vi "cDAQ Voltage - Finite Output.vi"() -> ()   [LabVIEW 2019]
doc: "This example demonstrates how to generate a finite amount of data from a buffer in your computer's memory."
uses:
  <vilib>/Utility/error.llb/DialogType.ctl
  <vilib>/DAQmx/write.llb/DAQmx Write (Analog 1D Wfm NChan NSamp).vi
  <vilib>/DAQmx/read.llb/DAQmx Read (Analog 1D DBL 1Chan NSamp).vi
  <vilib>/DAQmx/create/channels.llb/DAQmx Create Channel (AO-Voltage-Basic).vi
  <vilib>/DAQmx/configure/timing.llb/DAQmx Timing (Sample Clock).vi
  <vilib>/DAQmx/configure/trigger.llb/DAQmx Start Trigger (Digital Edge).vi
  <vilib>/DAQmx/configure/trigger.llb/DAQmx Start Trigger (Time).vi
  <vilib>/DAQmx/configure/trigger.llb/DAQmx Start Trigger (Analog Edge).vi
  <vilib>/DAQmx/miscellaneous.llb/DAQmx Fill In Error Info.vi
  <vilib>/DAQmx/configure/events/hardwareSignals.llb/DAQmx Export Signal (Most Signals).vi
  <vilib>/DAQmx/create/channels.llb/DAQmx Create Channel (AI-Voltage-Basic).vi
  <resource>/objmgr/daqmx.rc
  <vilib>/measure/NI_MABase.lvlib
panel:
  out "Waveform Graph 2":dbl[](graph)
  in  "physical channels":tag="cDAQ1Mod1/ai0"
  in  "Trigger Type":T1(tab)
  in  "Digital Start Trigger Edge":i32(ring)=10280 caption="Edge" items=["Rising"=10280, "Falling"=10171]
  in  "Digital Start Trigger Source":tag="/Dev1/PFI0" caption="Source"
  in  "Digital Pause Trigger Pause When":i32(ring)=10192 caption="Pause When" items=["High"=10192, "Low"=10214]
  in  "Digital Pause Trigger Source":tag="/Dev1/PFI0" caption="Source"
  in  "Analog Start Trigger Level":dbl caption="Level" format="%0.2f"
  in  "Analog Start Trigger Hysteresis":dbl caption="Hysteresis" format="%.2f"
  in  "Analog Start Trigger Slope":i32(ring)=10280 caption="Slope" items=["Rising"=10280, "Falling"=10171]
  in  "Analog Start Trigger Source":string="APFI0" caption="Source"
  in  "Analog Pause Trigger Source":string="APFI0" caption="Source"
  in  "Analog Pause Trigger Pause When":i32(ring)=10093 caption="Pause When" items=["Above Level"=10093, "Below Level"=10107]
  in  "Analog Pause Trigger Level":dbl caption="Level" format="%.2f"
  in  "When":timestamp
  in  "Select Time\nManually":bool
  in  "Output Array":T2(array[cluster])=[{"Waveform Type"=0, "Amplitude"=1.0, "Frequency"=10.0}] {"Frequency" format="%0.2p"; "Amplitude" format="%0.2p"; "Waveform Type" items=["Sine Wave", "Triangle Wave", "Square Wave", "Sawtooth Wave"]}
  in  "Number of Samples":i32=1000
  out "Waveform Graph":waveform(dbl)[](graph)=[{"t0"=timestamp(0 s since 1904-01-01), "dt"=0.001, "Y"=array[1000 elements]}]
  in  "Sample Rate":dbl=1000.0
  in  "Sample Clock Source":tag="OnboardClock"
  in  "Max Voltage":dbl=5.0
  in  "Min Voltage":dbl=-5.0
  in  "Physical Channel(s)":tag="cDAQ1Mod2/ao0"
  out "Actual Sample Rate":dbl=1000.0 format="%0.2f"
  # "Channel Settings"
  # "Output"
  # "Timing and Buffer Settings"
  # "Waveform Settings"
  # "Trigger Settings"
  # "The number of elements in the waveform array\nmust equal the number of channels in the task."
  # "To enable triggers, select a tab above, and configure the settings.\n\nNot all hardware supports all trigger types. Refer to your device documentation for more information."
  # "This trigger type is not supported in output tasks. \n\nRefer to your device documentation for more information on which triggers are supported."
  # "This trigger type is not supported in output tasks. \n\nRefer to your device documentation for more information on which triggers are supported."
  # "If time is not manually set, task will begin after 10 seconds"
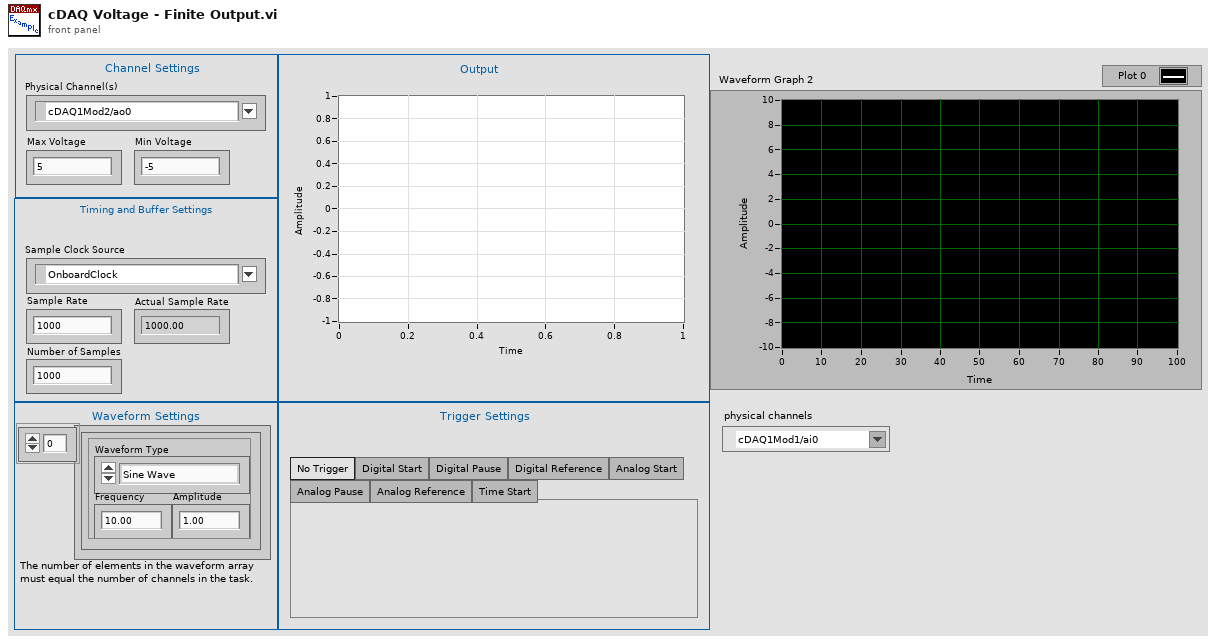
[diagram p1: front panel]
types:
  T1 = enum32{"No Trigger", "Digital Start", "Digital Pause", "Digital Reference", "Analog Start", "Analog Pause", "Analog Reference", "Time Start"}
  T2 = cluster{"Waveform Type":u16, "Amplitude":dbl, "Frequency":dbl}[]
  T3 = typedef "DialogType.ctl" = u16
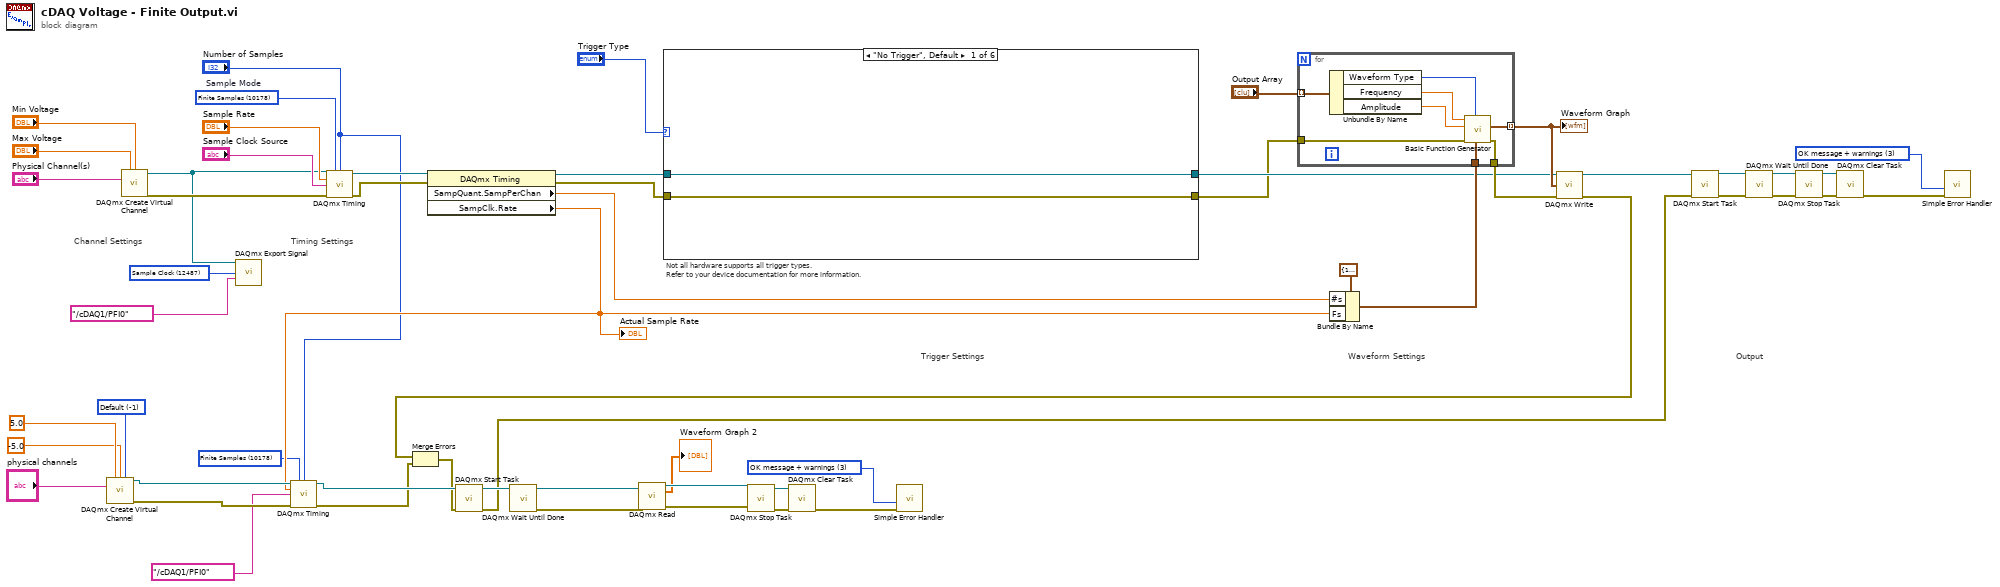
[diagram p0: block diagram]
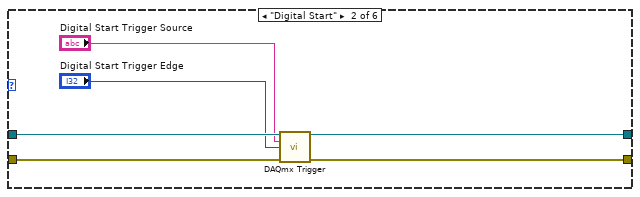
[diagram p2: hidden frame]
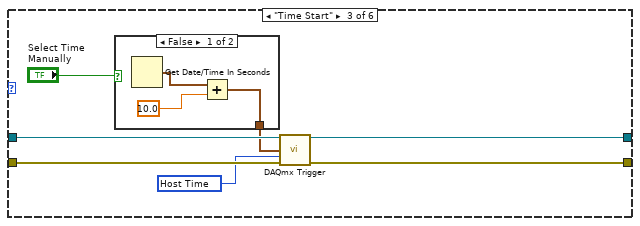
[diagram p3: hidden frame]
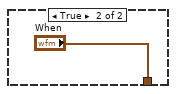
[diagram p4: hidden frame]
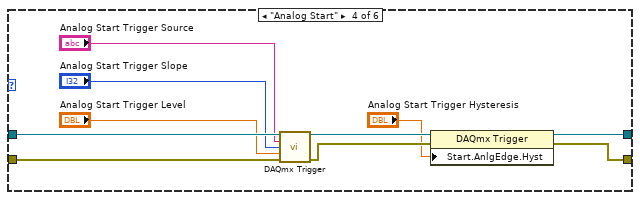
[diagram p5: hidden frame]
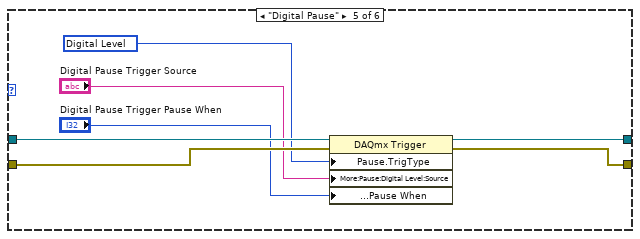
[diagram p6: hidden frame]
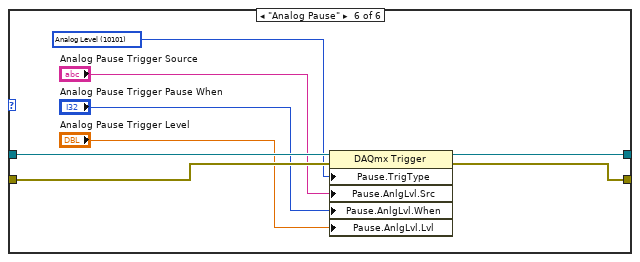
[diagram p7: hidden frame]
diagram:
  w8 = 10178 items=["Finite Samples"=10178, "Continuous Samples"=10123, "Hardware Timed Single Point"=12522] ("sample mode")
  w17 = T3 3 items=["no dialog", "OK message", "continue or stop message", "OK message + warnings", "continue/stop + warnings"] ("type of dialog (OK msg:1)")
  w22 = -1 items=["Default"=-1, "RSE"=10083, "NRSE"=10078, "Differential"=10106, "Pseudodifferential"=12529] ("input terminal configuration")
  w27 = 12487 items=["AI Convert Clock"=12484, "10MHz Reference Clock"=12536, "20MHz Timebase Clock"=12486, "Sample Clock"=12487, "Advance Trigger"=12488, "Reference Trigger"=12490, "Start Trigger"=12491, "Advance Complete Event"=12492, "AI Hold Complete Event"=12493, "Counter Output Event"=12494, "Change Detection Event"=12511, "Watchdog Timer Expired Event"=12512] ("signal")
  w34 = T3 3 items=["no dialog", "OK message", "continue or stop message", "OK message + warnings", "continue/stop + warnings"] ("type of dialog (OK msg:1)")
  w55 = 10178 items=["Finite Samples"=10178, "Continuous Samples"=10123, "Hardware Timed Single Point"=12522]  # Sample Mode
  # "Trigger Settings"
  # "Not all hardware supports all trigger types.\nRefer to your device documentation for more information."
  # "Output"
  # "Waveform Settings"
  # "Timing Settings"
  # "Channel Settings"
  n1 = call-poly <vilib>:"DAQmx Create Virtual Channel.vi"("maximum value"=5.0, "minimum value"=-5.0, "input terminal configuration"=w22, "physical channels"="physical channels") -> ("task out"=w16:refnum<k21>, "error out"=w12:errorcluster)  [unwired: 10 in]
  n2 = call-poly <vilib>:"DAQmx Create Virtual Channel.vi"("maximum value"="Max Voltage", "minimum value"="Min Voltage", "physical channels"="Physical Channel(s)") -> ("task out"=w28:refnum<k21>, "error out"=w54:errorcluster)  [unwired: 11 in]
  n3 = call-poly <vilib>:"DAQmx Export Signal.vi"("task/channels in"=w28, "signal"=w27, "output terminal"=tag "/cDAQ1/PFI0") -> ()  [unwired: 11 in, 2 out]
  n4 = call-poly <vilib>:"DAQmx Timing.vi"("task/channels in"=w28, "sample mode"=w55, "samples per channel"="Number of Samples", "rate"="Sample Rate", "source"="Sample Clock Source", "error in"=w54) -> ("task out"=w57:refnum<k21>, "error out"=w56:errorcluster)  [unwired: 8 in]
  n5 = property class="DAQmx Timing"(reference=w57, error in=w56) -> (reference out=w29:refnum<k21>, error out=w30:errorcluster, "SampQuant.SampPerChan"=w39:dbl, "SampClk.Rate"=w9:dbl)
  "Actual Sample Rate" <- w9
  n6 = call-poly <vilib>:"DAQmx Timing.vi"("task/channels in"=w16, "sample mode"=w8, "samples per channel"="Number of Samples", "rate"=w9, "source"=tag "/cDAQ1/PFI0", "error in"=w12) -> ("task out"=w15:refnum<k21>, "error out"=w3:errorcluster)  [unwired: 8 in]
  n7 = case shown="\"No Trigger\", Default" "Trigger Type" {
    tunnel: w29 -> [w59 w65 w72 w86 w93 w101]
    tunnel: w30 -> [w58 w64 w71 w85 w90 w98]
    tunnel: [w59 w63 w70 w83 w92 w100] -> w32
    tunnel: [w58 w62 w69 w82 w91 w99] -> w31
    frame "No Trigger", Default {
    }
    frame "Digital Start" {
      n8 = call-poly <vilib>:"DAQmx Trigger.vi"("task/channels in"=w65, "source"="Digital Start Trigger Source", "edge"="Digital Start Trigger Edge", "error in"=w64) -> ("task out"=w63:refnum<k21>, "error out"=w62:errorcluster)  [unwired: 10 in]
    }
    frame "Time Start" {
      w68 = 16126 items=["Host Time"=16126, "I/O Device Time"=16127] ("timescale")
      n9 = case shown="False" "Select Time\nManually" {
        tunnel: [w74 "When"] -> w66
        frame False {
          n10 = Get Date/Time In Seconds() -> (seconds since 1Jan1904=w75:timestamp)
          n11 = Add(x=w75, y=10.0) -> (x+y=w74:timestamp)
        }
        frame True {
        }
      }
      n12 = call-poly <vilib>:"DAQmx Trigger.vi"("task/channels in"=w72, "when"=w66, "timescale"=w68, "error in"=w71) -> ("task out"=w70:refnum<k21>, "error out"=w69:errorcluster)  [unwired: 10 in]
    }
    frame "Analog Start" {
      n13 = call-poly <vilib>:"DAQmx Trigger.vi"("task/channels in"=w86, "source"="Analog Start Trigger Source", "slope"="Analog Start Trigger Slope", "level"="Analog Start Trigger Level", "error in"=w85) -> ("task out"=w81:refnum<k21>, "error out"=w80:errorcluster)  [unwired: 9 in]
      n14 = property class="DAQmx Trigger"(reference=w81, error in=w80, "Start.AnlgEdge.Hyst"="Analog Start Trigger Hysteresis") -> (reference out=w83:refnum<k21>, error out=w82:errorcluster)
    }
    frame "Digital Pause" {
      w89 = 10152 items=["Analog Level"=10101, "Analog Window"=10103, "Digital Level"=10152, "Digital Pattern"=10398, "None"=10230] ("Pause.TrigType")
      n15 = property class="DAQmx Trigger"(reference=w93, error in=w90, "Pause.TrigType"=w89, "More:Pause:Digital Level:Source"="Digital Pause Trigger Source", "More:Pause:Digital Level:Pause When"="Digital Pause Trigger Pause When") -> (reference out=w92:refnum<k21>, error out=w91:errorcluster)
    }
    frame "Analog Pause" {
      w97 = 10101 items=["Analog Level"=10101, "Analog Window"=10103, "Digital Level"=10152, "Digital Pattern"=10398, "None"=10230] ("Pause.TrigType")
      n16 = property class="DAQmx Trigger"(reference=w101, error in=w98, "Pause.TrigType"=w97, "Pause.AnlgLvl.Src"="Analog Pause Trigger Source", "Pause.AnlgLvl.When"="Analog Pause Trigger Pause When", "Pause.AnlgLvl.Lvl"="Analog Pause Trigger Level") -> (reference out=w100:refnum<k21>, error out=w99:errorcluster)
    }
  }
  n17 = Bundle By Name(cluster=cluster{"Fs":dbl, "#s":dbl} {"Fs"=1000.0, "#s"=1000.0} ("sampling info"), "#s"=w39, "Fs"=w9) -> (w46:cluster{"Fs":dbl, "#s":dbl})
  n18 = for {
    tunnel: w31 -> [w109]
    tunnel: w46 -> [w108]
    tunnel: [w107] -> w44
    tunnel: "Output Array" -> [w106] mode=indexing
    tunnel: [w102] -> w42 mode=indexing
    n19 = Unbundle By Name(w106) -> ("Waveform Type"=w105:u16, "Frequency"=w104:dbl, "Amplitude"=w103:dbl)
    n20 = call <vilib>:"Basic Function Generator.vi"("sampling info"=w108, "signal type"=w105, "error in (no error)"=w109, "amplitude"=w103, "frequency"=w104) -> ("error out"=w107:errorcluster, "signal out"=w102:waveform(dbl))  [unwired: 4 in, 1 out]
  }
  "Waveform Graph" <- w42
  n21 = call-poly <vilib>:"DAQmx Write.vi"("task/channels in"=w32, "data"=w42, "error in"=w44) -> ("task out"=w45:refnum<k21>, "error out"=w4:errorcluster)  [unwired: 10 in, 1 out]
  n22 = Merge Errors(w4, w3) -> (w2:errorcluster)
  n23 = call <vilib>:"DAQmx Start Task.vi"("task/channels in"=w15, "error in"=w2) -> ("task out"=w20:refnum<k21>, "error out"=w1:errorcluster)  [unwired: 12 in]
  n24 = call <vilib>:"DAQmx Wait Until Done.vi"("task/channels in"=w20) -> ("task out"=w14:refnum<k21>, "error out"=w11:errorcluster)  [unwired: 13 in]
  n25 = call-poly <vilib>:"DAQmx Read.vi"("task/channels in"=w14, "error in"=w11) -> ("task out"=w13:refnum<k21>, "data"=→"Waveform Graph 2":dbl[], "error out"=w10:errorcluster)  [unwired: 11 in]
  n26 = call <vilib>:"DAQmx Stop Task.vi"("task/channels in"=w13, "error in"=w10) -> ("task out"=w19:refnum<k21>, "error out"=w18:errorcluster)  [unwired: 12 in]
  n27 = call <vilib>:"DAQmx Clear Task.vi"("task in"=w19, "error in"=w18) -> ("error out"=w21:errorcluster)  [unwired: 13 in]
  n28 = call <vilib>:"Simple Error Handler.vi"("type of dialog (OK msg:1)"=w17, "error in (no error)"=w21) -> ()  [unwired: 3 in, 5 out]
  n29 = call <vilib>:"DAQmx Start Task.vi"("task/channels in"=w45, "error in"=w1) -> ("task out"=w41:refnum<k21>, "error out"=w40:errorcluster)  [unwired: 12 in]
  n30 = call <vilib>:"DAQmx Wait Until Done.vi"("task/channels in"=w41, "error in"=w40) -> ("task out"=w36:refnum<k21>, "error out"=w35:errorcluster)  [unwired: 12 in]
  n31 = call <vilib>:"DAQmx Stop Task.vi"("task/channels in"=w36, "error in"=w35) -> ("task out"=w38:refnum<k21>, "error out"=w37:errorcluster)  [unwired: 12 in]
  n32 = call <vilib>:"DAQmx Clear Task.vi"("task in"=w38, "error in"=w37) -> ("error out"=w53:errorcluster)  [unwired: 13 in]
  n33 = call <vilib>:"Simple Error Handler.vi"("type of dialog (OK msg:1)"=w34, "error in (no error)"=w53) -> ()  [unwired: 3 in, 5 out]
